vi "integrate.vi"(9 "Longitud":i32, 10 "inicio":i32, 11 "Array":u32[](array[numeric])) -> (3 "result":dbl format="%0.4f")   [LabVIEW 2021]
uses:
  <vilib>/Analysis/2dsp.llb/Integral Method.ctl
  <vilib>/Analysis/8numeric.llb/1D Numeric Integration.vi
  <vilib>/Analysis/NI_AALPro.lvlib
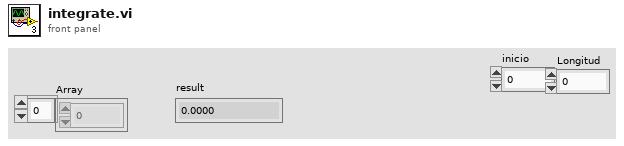
[diagram p1: front panel]
types:
  T1 = typedef "NI_AALPro.lvlib/Integral Method.ctl" = i32
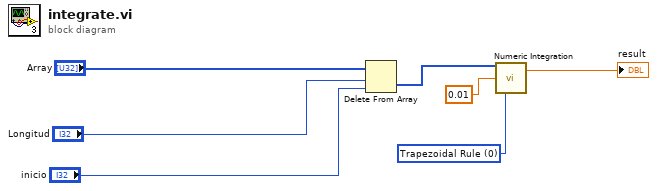
[diagram p0: block diagram]
diagram:
  w7 = T1 0 items=["Trapezoidal Rule", "Simpson's Rule", "Simpson's 3/8 Rule", "Bode Rule"] ("integration method")
  n1 = Delete From Array(array="Array", length="Longitud", index="inicio") -> (deleted portion=w1:u32[])  [unwired: 1 out]
  n2 = call-poly <vilib>:"Numeric Integration.vi"("integration method"=w7, "dt"=0.01, "Input Array"=w1) -> ("result"=→"result":dbl)  [unwired: 1 out]
